vi "UR LabVIEW SFTP Interface1.vi"() -> ()   [LabVIEW 2019]
uses:
  LabSSH Library/SFTP Library/Connection Info..cluster.ctl
  LabSSH Library/SFTP Library/Password..cluster.ctl
  LabSSH Library/SFTP Library/connect_password.vi
  LabSSH Library/SFTP Library/LabSFTP.lvlib
panel:
  in  "Multicolumn Listbox":i32(listbox)
  out "Array 2":string[](array[string])
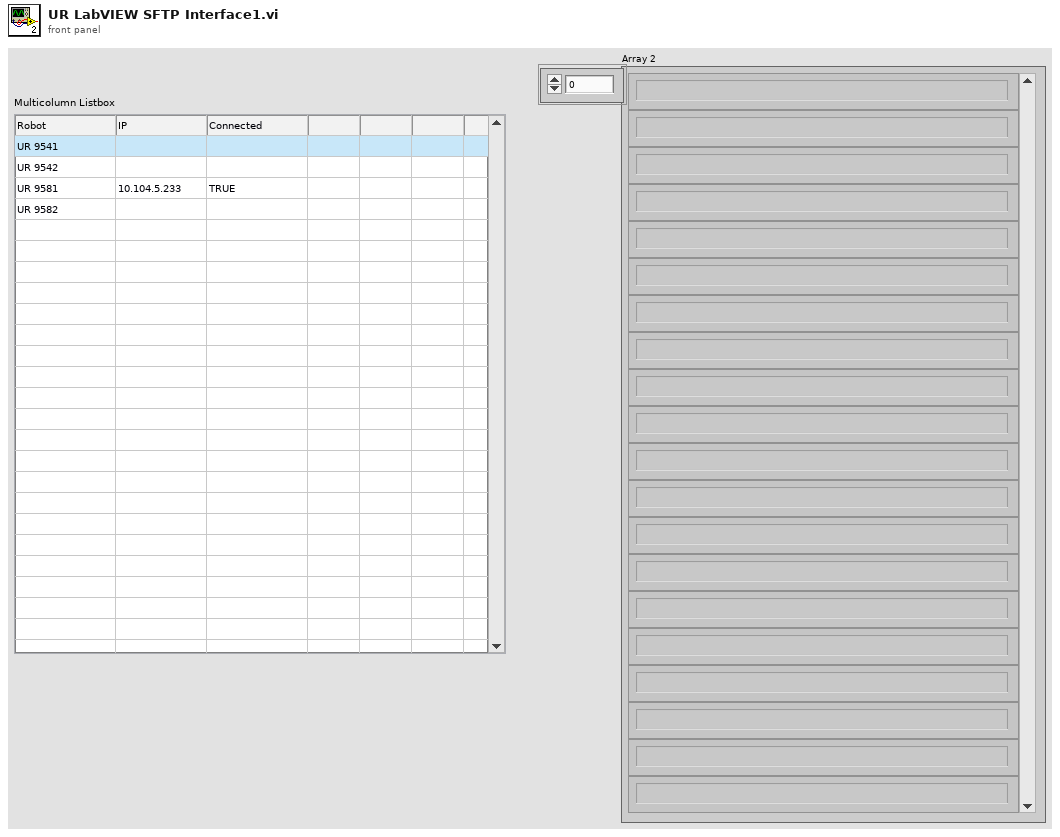
[diagram p1: front panel]
types:
  T1 = typedef "LabSFTP.lvlib/Password..cluster.ctl" = cluster{"Password":string}
  T2 = typedef "LabSFTP.lvlib/Connection Info..cluster.ctl" = cluster{"Remote":string, "Username":string, "Port (22)":i32}
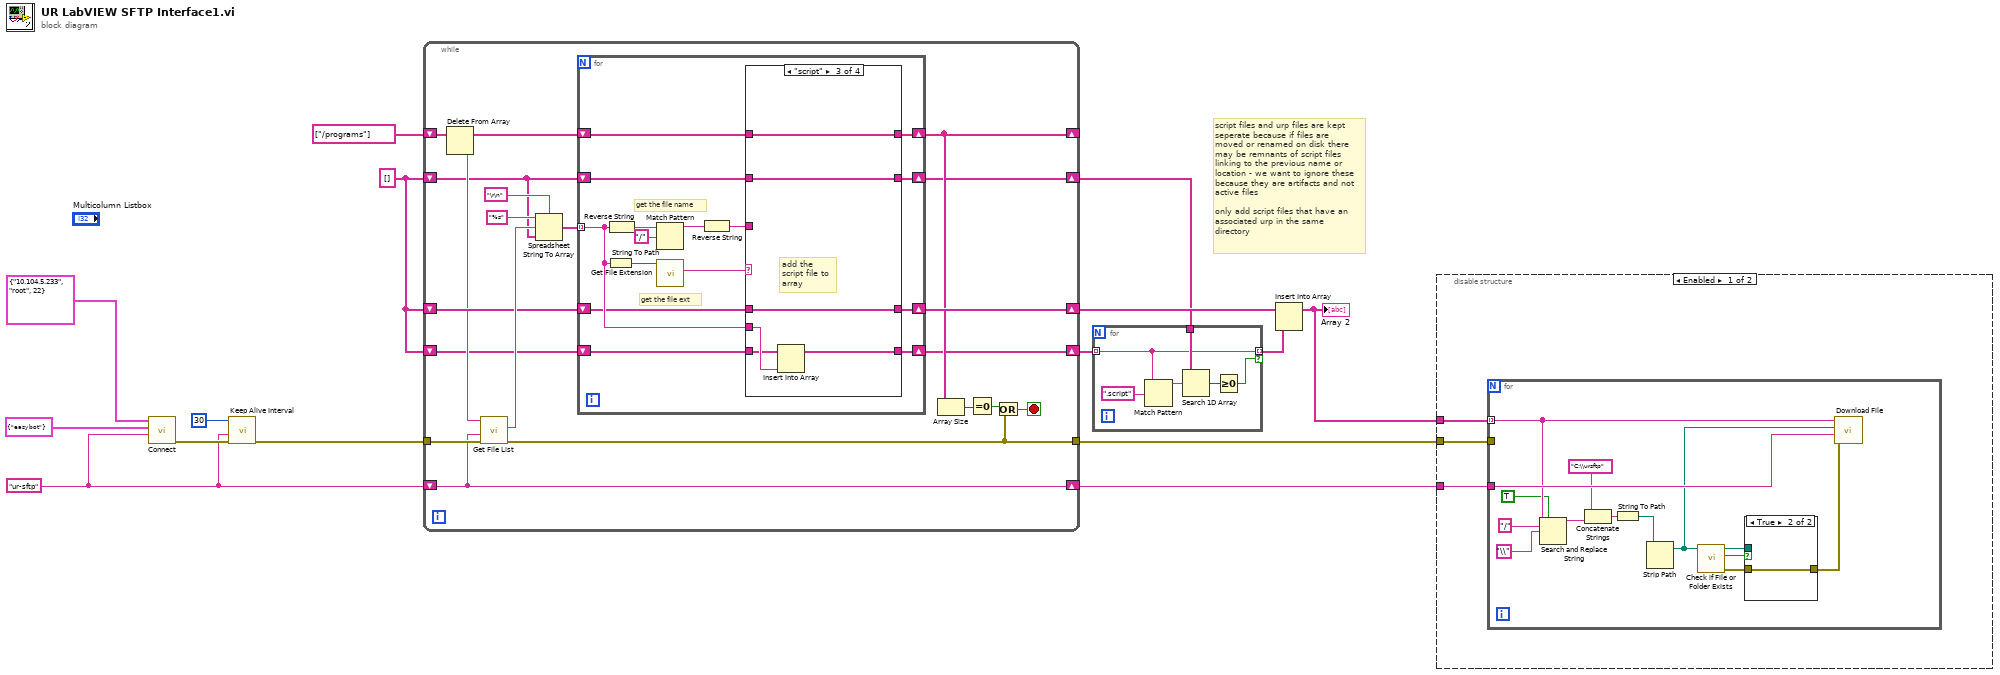
[diagram p0: block diagram]
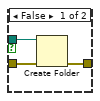
[diagram p2: hidden frame]
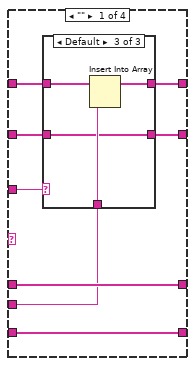
[diagram p4: hidden frame]
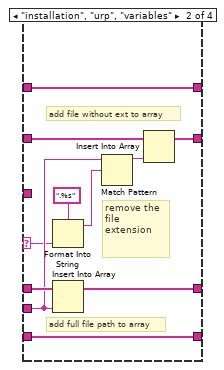
[diagram p7: hidden frame]
diagram:
  w1 = string[] []
  w11 = "ur-sftp" ("Connection Name")
  # "script files and urp files are kept seperate because if files are moved or renamed on disk there may be remnants of script files linking to the previous name or location - we want to ignore these because they are artifacts and not active files\n\nonly add script files that have an associated urp in the same directory"
  n1 = call-poly "Connect.vi"("Connection Name"=w11, "Password"=T1 {"Password"="easybot"}, "Connection Info."=T2 {"Remote"="10.104.5.233", "Username"="root", "Port (22)"=22}) -> ("error out"=w12:errorcluster)  [unwired: 6 in, 2 out]
  n2 = call "Keep Alive Interval.vi"("error in (no error)"=w12, "Connection Name"=w11, "Keep Alive Interval (s)"=30) -> ("error out"=w9:errorcluster)  [unwired: 8 in]
  n3 = while {
    shift-right: [w30] -> w5
    shift-left: w1 -> [w29]
    shift-right: [w25] -> _
    shift-left: string[] ["/programs"] -> [w28]
    tunnel: w9 -> [w35]
    tunnel: [w22] -> w8
    shift-right: [w20] -> w7
    shift-left: w11 -> [w20]
    shift-right: [w19] -> w6
    shift-left: w1 -> [w18]
    shift-right: [w17] -> w3
    shift-left: w1 -> [w16]
    stop <- w21 stop-if-true
    n4 = Delete From Array(array=w28) -> (deleted portion=w26:string, array with subset deleted=w27:string[])  [unwired: 2 in]
    n5 = call "Get File List.vi"("error in (no error)"=w35, "Connection Name"=w20, "Remote Path"=w26) -> ("error out"=w22:errorcluster, "File List"=w34:string)  [unwired: 6 in, 1 out]
    n6 = Spreadsheet String To Array(delimiter (Tab)="\r\n", format string="%s", spreadsheet string=w34, array type (2D Dbl)=w16) -> (array=w31:string[])
    n7 = for {
      tunnel: w31 -> [w44] mode=indexing
      shift-right: [w43] -> w30
      shift-left: w29 -> [w42]
      shift-right: [w41] -> w25
      shift-left: w27 -> [w40]
      shift-right: [w39] -> w19
      shift-left: w18 -> [w38]
      shift-right: [w37] -> w17
      shift-left: w16 -> [w36]
      # "get the file ext"
      # "get the file name"
      n8 = String To Path(string=w44) -> (path=w48:path)
      n9 = Reverse String(1:w44) -> (0:w50:string)
      n10 = Match Pattern(string=w50, regular expression="/") -> (before substring=w47:string)  [unwired: 1 in, 3 out]
      n11 = call <vilib>:"Get File Extension.vi"("file"=w48) -> ("lowercase file extension"=w46:string)  [unwired: 6 in, 4 out]
      n12 = Reverse String(1:w47) -> (0:w45:string)
      n13 = case shown="\"script\"" w46 {
        selector: w46 -> [_ w69 _ _]
        tunnel: w45 -> [w57 _ _ _]
        tunnel: w44 -> [w56 w71 w83 _]
        tunnel: [w58 w77 w81 w87] -> w43
        tunnel: w42 -> [w58 w76 w81 w87]
        tunnel: [w55 w75 w82 w86] -> w41
        tunnel: w40 -> [w54 w75 w82 w86]
        tunnel: [w53 w74 w80 w85] -> w39
        tunnel: w38 -> [w53 w74 w79 w85]
        tunnel: [w51 w73 w78 w84] -> w37
        tunnel: w36 -> [w52 w72 w78 w84]
        frame "" {
          n14 = case shown="Default" w57 {
            tunnel: w56 -> [_ _ w66]
            tunnel: [w60 w62 w65] -> w55
            tunnel: w54 -> [w60 w62 w64]
            tunnel: w52 -> [w59 w61 w63]
            tunnel: [w59 w61 w63] -> w51
            frame "", ".", ".." {
              # "invalid folder"
            }
            frame "usbdisk".."usbdisk~" {
              # "invalid folder"
            }
            frame Default {
              n15 = Insert Into Array(array=w64, new element=w66) -> (w65:string[])  [unwired: 1 in]
            }
          }
        }
        frame "installation", "urp", "variables" {
          # "remove the file extension"
          # "add file without ext to array"
          # "add full file path to array"
          n16 = Format Into String(format string=".%s", w69) -> (resulting string=w68:string)  [unwired: 2 in, 1 out]
          n17 = Insert Into Array(array=w76, new element=w71) -> (w77:string[])  [unwired: 1 in]
          n18 = Match Pattern(string=w71, regular expression=w68) -> (before substring=w70:string)  [unwired: 1 in, 3 out]
          n19 = Insert Into Array(array=w72, new element=w70) -> (w73:string[])  [unwired: 1 in]
        }
        frame "script" {
          # "add the script file to array"
          n20 = Insert Into Array(array=w79, new element=w83) -> (w80:string[])  [unwired: 1 in]
        }
        frame Default {
        }
      }
    }
    n21 = Array Size(array=w25) -> (size(s)=w24:i32)
    n22 = Equal To 0?(x=w24) -> (x = 0?=w23:bool)
    n23 = Or(x=w23, y=w22) -> (x .or. y?=w21:bool)
  }
  n24 = for {
    tunnel: w6 -> [w90] mode=indexing
    tunnel: [w90] -> w4 mode=indexing if=w91
    tunnel: w3 -> [w93]
    n25 = Match Pattern(string=w90, regular expression=".script") -> (before substring=w88:string)  [unwired: 1 in, 3 out]
    n26 = Search 1D Array(1D array=w93, element=w88) -> (index of element=w92:i32)  [unwired: 1 in]
    n27 = Greater Or Equal To 0?(x=w92) -> (x >= 0?=w91:bool)
  }
  n28 = Insert Into Array(array=w5, new element=w4) -> (w2:string[])  [unwired: 1 in]
  "Array 2" <- w2
  n29 = disable-structure shown="Enabled" {
    disable-tunnel: w8 -> [w96 _]
    disable-tunnel: w7 -> [w95 _]
    disable-tunnel: w2 -> [w94 _]
    frame Enabled {
      n30 = for {
        tunnel: w96 -> [_]
        tunnel: w95 -> [w110]
        tunnel: w94 -> [w109] mode=indexing
        n31 = Search and Replace String(replace all?=TRUE ("replace all? (F)"), input string=w109, search string="/", replace string="\\" ("replace string (\"\")")) -> (result string=w105:string)  [unwired: 4 in, 3 out]
        n32 = Concatenate Strings("C:\\ursftp" ("string"), w105) -> (w103:string)
        n33 = String To Path(string=w103) -> (path=w102:path)
        n34 = Strip Path(path=w102) -> (stripped path=w97:path)  [unwired: 1 out]
        n35 = call <vilib>:"Check if File or Folder Exists.vi"("path"=w97) -> ("error out"=w99:errorcluster, "file or folder exists?"=w101:bool, "dup path"=w100:path)  [unwired: 8 in]
        n36 = case shown="True" w101 {
          tunnel: w100 -> [w113 _]
          tunnel: w99 -> [w112 w114]
          tunnel: [w111 w114] -> w98
          frame False {
            n37 = Create Folder(path (use dialog)=w113, error in=w112) -> (error out=w111:errorcluster)  [unwired: 1 in, 2 out]
          }
          frame True {
          }
        }
        n38 = call "Download File.vi"("error in (no error)"=w98, "Connection Name"=w110, "Local File Path"=w97, "Remote File Path"=w109) -> ()  [unwired: 6 in, 2 out]
      }
    }
    frame Disabled {
    }
  }
